vi "SubVI_SingleSymbolWrite.vi"(8 "error in":errorcluster, 9 "WData":variant, 10 "SymbolName":string, 11 "Handle In":u32) -> (0 "error out":errorcluster, 1 "bHasMatched":bool, 2 "Write Status":bool, 3 "Handle Out":u32)   [LabVIEW 2022 SP3, in "ADS_Library.lvlib"]
uses:
  ADS_Library.lvlib
  <userlib>/Beckhoff-LabVIEW-Interface/_DependsOn/Base/TypeResolver/Set TypeResolver.vi
  <userlib>/Beckhoff-LabVIEW-Interface/_DependsOn/Base/Write/Write Sync.vi
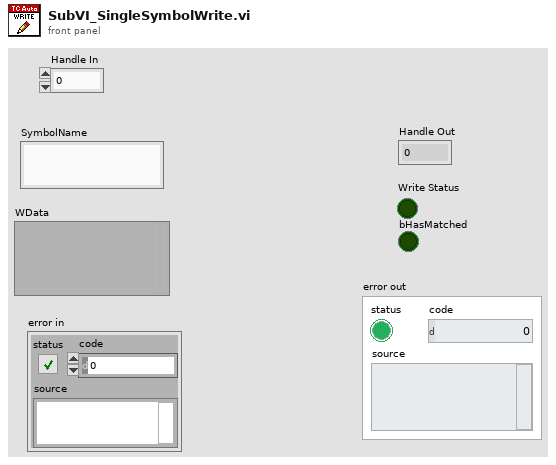
[diagram p1: front panel]
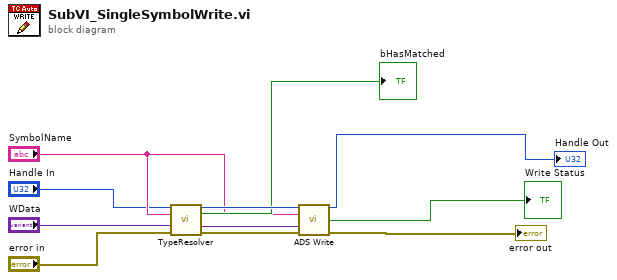
[diagram p0: block diagram]
diagram:
  n1 = call-poly <userlib>:"TypeResolver.vi"("Handle"="Handle In", "SymbolName"="SymbolName", "WData"="WData", "error in"="error in") -> ("Handle"=w8:u32, "bHasMatched"=→"bHasMatched":bool, "ADSWData"=w9:variant, "error out"=w10:errorcluster)  [unwired: 8 in]
  n2 = call-poly <userlib>:"ADS Write.vi"("Handle"=w8, "SymbolName"="SymbolName", "Ads Write Data"=w9, "error in (no error)"=w10) -> ("Handle"=→"Handle Out":u32, "Write Status"=→"Write Status":bool, "error out"=→"error out":errorcluster)  [unwired: 8 in, 1 out]
